vi "DCA Convert Limits Cluster.vi"(4 "Fields Names":string[](array[string]), 5 "Conversion":enum16{"Cluster - HTML", "HTML - Cluster"}(ring), 7 "Limits Key Array In":T6, 8 "Limits Cluster In":T1[](array[typedef])) -> (1 "Limits Cluster Out":T1[](array[typedef]), 2 "Limits HTML Out":string)   [LabVIEW 2011]
uses:
  ITK EXT/utils/keyedarr.llb/Keyed Array.ctl
  TypeDefs/DCA Limit.ctl
  TypeDefs/DCA Limit Quantity.ctl
  TypeDefs/DCA Limit Comparison.ctl
  TypeDefs/DCA Limit Operation.ctl
  Test Referential Limit.ctl
  ITK EXT/utils/strutil.llb/Case Matching.ctl
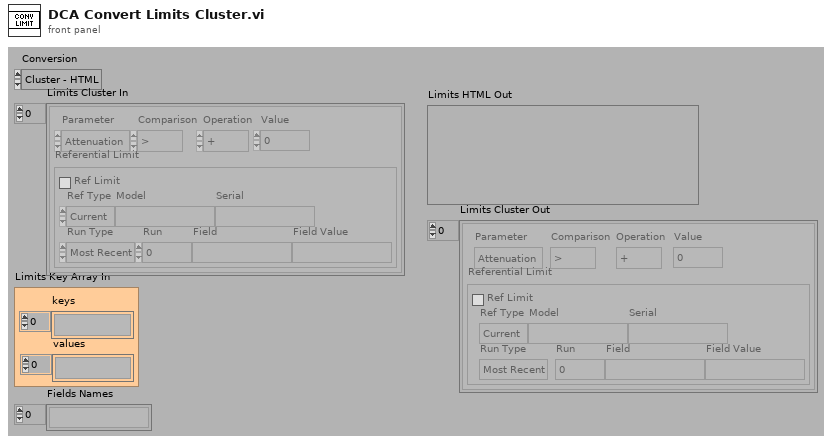
[diagram p1: front panel]
types:
  T1 = typedef "DCA Limit.ctl" = cluster{"Parameter":T2, "Comparison":T3, "Operation":T4, "Value":dbl, "Referential Limit":T5}
  T2 = typedef "DCA Limit Quantity.ctl" = enum16{"Attenuation", "Zin", "Zout", "R1", "R2", "R3", "Rab", "Rac", "Rbc"}
  T3 = typedef "DCA Limit Comparison.ctl" = enum16{">", ">=", "<", "<="}
  T4 = typedef "DCA Limit Operation.ctl" = enum16{"+", "-"}
  T5 = typedef "Test Referential Limit.ctl" = cluster{"Ref Limit":bool, "Ref Type":enum16{"Current", "Specify"}, "Model":string, "Serial":string, "Run Type":enum16{"Most Recent", "Run #", "Match Field"}, "Run":i32, "Field":string, "Field Value":string}
  T6 = typedef "Keyed Array.ctl" = cluster{"keys":string[], "values":string[]}
  T7 = typedef "Case Matching.ctl" = enum16{"a != A", "a == A", "system"}
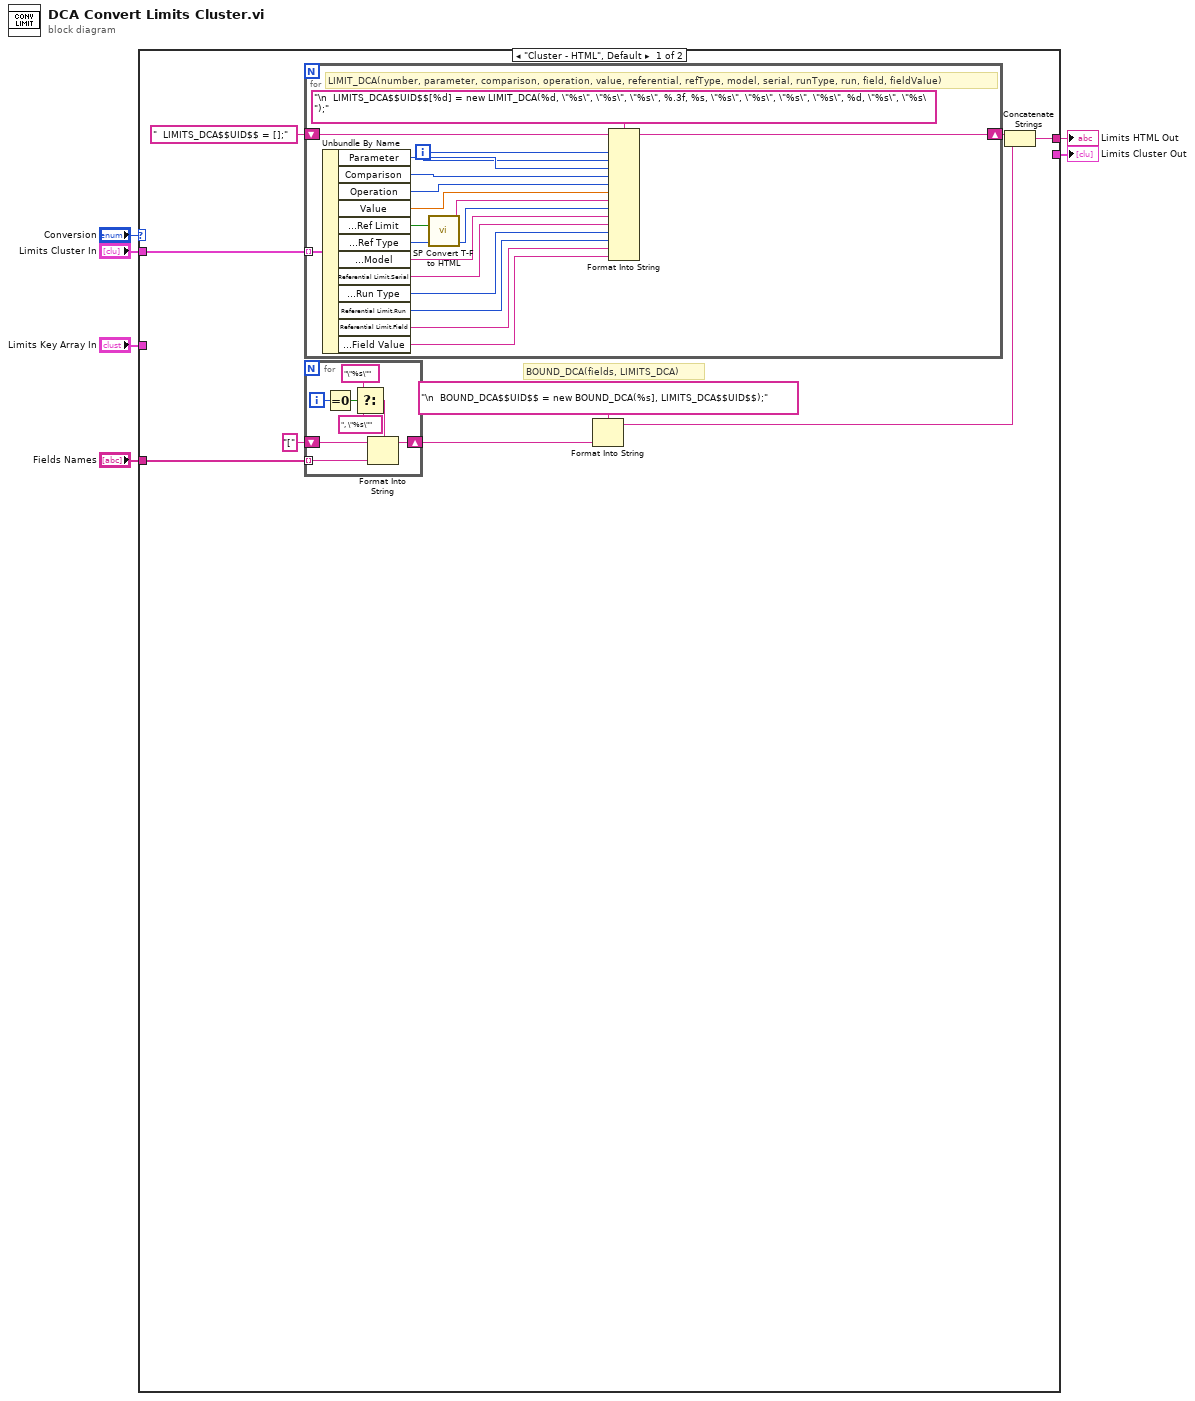
[diagram p0: block diagram]
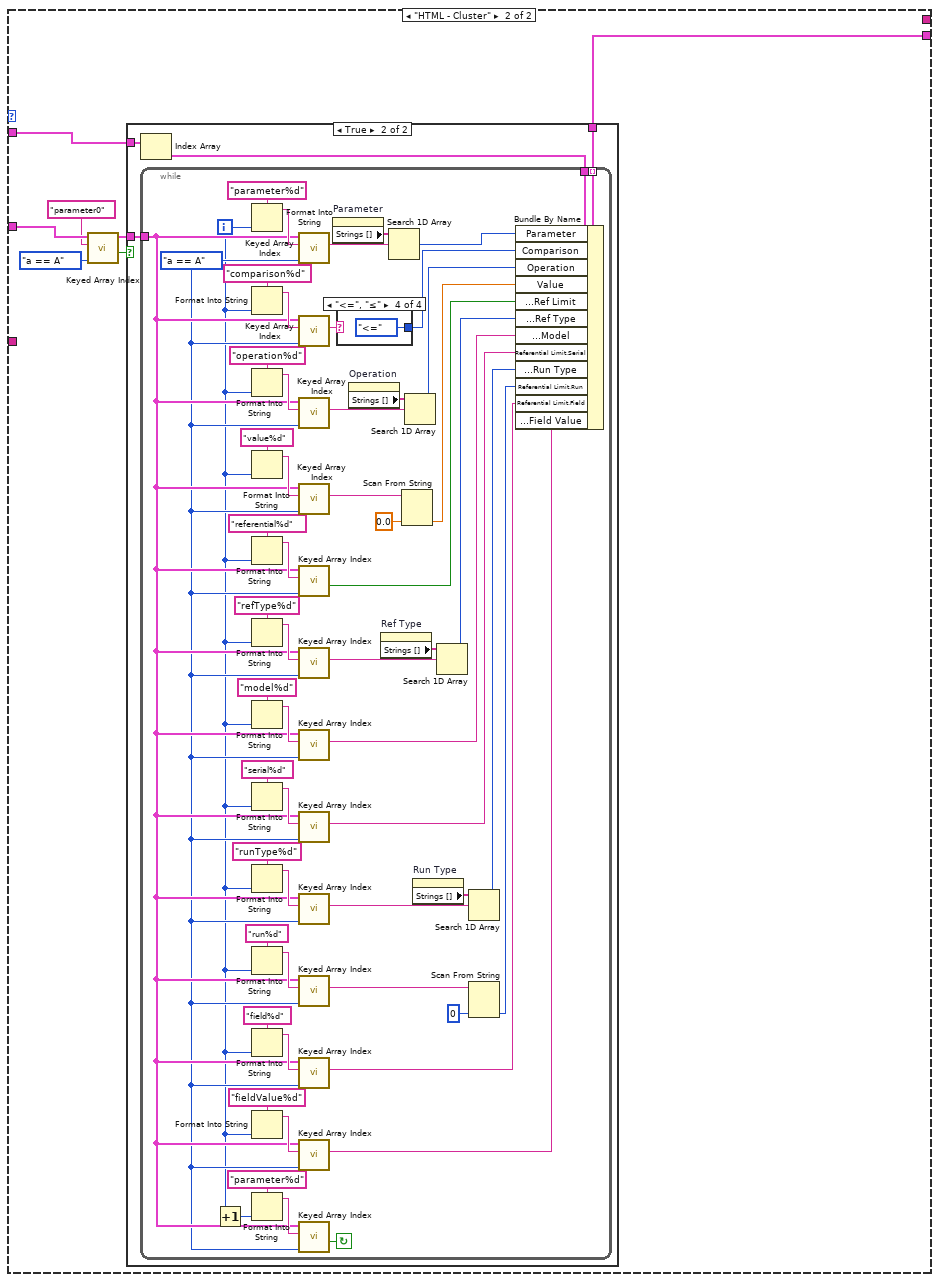
[diagram p2: hidden frame]
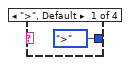
[diagram p4: hidden frame]
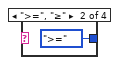
[diagram p5: hidden frame]
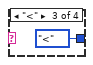
[diagram p6: hidden frame]
diagram:
  n1 = case shown="\"Cluster - HTML\", Default" "Conversion" {
    tunnel: "Limits Cluster In" -> [w15 w48]
    tunnel: "Limits Key Array In" -> [_ w46]
    tunnel: [w13 _] -> w3
    tunnel: [_ w47] -> w2
    tunnel: "Fields Names" -> [w10 _]
    frame "Cluster - HTML", Default {
      # "BOUND_DCA(fields, LIMITS_DCA)"
      n2 = for {
        tunnel: w15 -> [w41] mode=indexing
        shift-right: [w40] -> w12
        shift-left: "  LIMITS_DCA$$UID$$ = [];" ("format string") -> [w24]
        i -> [w25]
        # "LIMIT_DCA(number, parameter, comparison, operation, value, referential, refType, model, serial, runType, run, field, fieldValue)"
        n3 = Unbundle By Name(w41) -> ("Parameter"=w37:T2, "Comparison"=w36:T3, "Operation"=w35:T4, "Value"=w34:dbl, "Referential Limit.Ref Limit"=w38:bool, "Referential Limit.Ref Type"=w32:enum16{"Current", "Specify"}, "Referential Limit.Model"=w31:string, "Referential Limit.Serial"=w30:string, "Referential Limit.Run Type"=w29:enum16{"Most Recent", "Run #", "Match Field"}, "Referential Limit.Run"=w28:i32, "Referential Limit.Field"=w27:string, "Referential Limit.Field Value"=w26:string)
        n4 = call "SP Convert T-F to HTML.vi"("(T/F)"=w38) -> ("HTML (true/false)"=w33:string)  [unwired: 10 out]
        n5 = Format Into String(format string="\n  LIMITS_DCA$$UID$$[%d] = new LIMIT_DCA(%d, \"%s\", \"%s\", \"%s\", %.3f, %s, \"%s\", \"%s\", \"%s\", \"%s\", %d, \"%s\", \"%s\");", initial string=w24, w25, w25, w37, w36, w35, w34, w33, w32, w31, w30, w29, w28, w27, w26) -> (resulting string=w40:string)  [unwired: 1 in, 1 out]
      }
      n6 = for {
        shift-right: [w16] -> w8
        shift-left: "[" ("format string") -> [w23]
        tunnel: w10 -> [w17] mode=indexing
        i -> [w22]
        n7 = Equal To 0?(x=w22) -> (x = 0?=w21:bool)
        n8 = Select(t="\"%s\"" ("format string"), s=w21, f=", \"%s\"" ("format string")) -> (s? t:f=w18:string)
        n9 = Format Into String(format string=w18, initial string=w23, w17) -> (resulting string=w16:string)  [unwired: 1 in, 1 out]
      }
      n10 = Format Into String(format string="\n  BOUND_DCA$$UID$$ = new BOUND_DCA(%s], LIMITS_DCA$$UID$$);", w8) -> (resulting string=w7:string)  [unwired: 2 in, 1 out]
      n11 = Concatenate Strings(w12, w7) -> (w13:string)
    }
    frame "HTML - Cluster" {
      n12 = call "Keyed Array Index.vi"("case matching (sensitive)"=Case_Matching."a == A", "key"="parameter0", "array in"=w46) -> ("valid key"=w43:bool, "duplicate array"=w45:T6)  [unwired: 1 in, 2 out]
      n13 = case shown="True" w43 {
        tunnel: w48 -> [_ w52]
        tunnel: [_ w51] -> w47
        tunnel: w45 -> [_ w50]
        frame False {
        }
        frame True {
          n14 = Index Array(array=w52) -> (element=w49:T1)  [unwired: 1 in]
          n15 = while {
            tunnel: w49 -> [w110]
            tunnel: [w109] -> w51 mode=indexing
            tunnel: w50 -> [w59]
            i -> [w57]
            stop <- w67 continue-if-true
            w58 = Case_Matching."a == A" ("case matching (sensitive)")
            n16 = Increment(x=w57) -> (x+1=w68:i32)
            n17 = Format Into String(format string="parameter%d", w57) -> (resulting string=w107:string)  [unwired: 2 in, 1 out]
            n18 = Format Into String(format string="comparison%d", w57) -> (resulting string=w106:string)  [unwired: 2 in, 1 out]
            n19 = Format Into String(format string="operation%d", w57) -> (resulting string=w103:string)  [unwired: 2 in, 1 out]
            n20 = Format Into String(format string="value%d", w57) -> (resulting string=w60:string)  [unwired: 2 in, 1 out]
            n21 = Format Into String(format string="referential%d", w57) -> (resulting string=w102:string)  [unwired: 2 in, 1 out]
            n22 = Format Into String(format string="refType%d", w57) -> (resulting string=w99:string)  [unwired: 2 in, 1 out]
            n23 = Format Into String(format string="model%d", w57) -> (resulting string=w98:string)  [unwired: 2 in, 1 out]
            n24 = Format Into String(format string="serial%d", w57) -> (resulting string=w95:string)  [unwired: 2 in, 1 out]
            n25 = Format Into String(format string="runType%d", w57) -> (resulting string=w94:string)  [unwired: 2 in, 1 out]
            n26 = Format Into String(format string="run%d", w57) -> (resulting string=w91:string)  [unwired: 2 in, 1 out]
            n27 = Format Into String(format string="field%d", w57) -> (resulting string=w90:string)  [unwired: 2 in, 1 out]
            n28 = Format Into String(format string="fieldValue%d", w57) -> (resulting string=w87:string)  [unwired: 2 in, 1 out]
            n29 = Format Into String(format string="parameter%d", w68) -> (resulting string=w70:string)  [unwired: 2 in, 1 out]
            n30 = call "Keyed Array Index.vi"("case matching (sensitive)"=w58, "key"=w107, "array in"=w59) -> ("value"=w65:string)  [unwired: 1 in, 3 out]
            n31 = call "Keyed Array Index.vi"("case matching (sensitive)"=w58, "key"=w106, "array in"=w59) -> ("value"=w54:string)  [unwired: 1 in, 3 out]
            n32 = call "Keyed Array Index.vi"("case matching (sensitive)"=w58, "key"=w103, "array in"=w59) -> ("value"=w85:string)  [unwired: 1 in, 3 out]
            n33 = call "Keyed Array Index.vi"("case matching (sensitive)"=w58, "key"=w60, "array in"=w59) -> ("value"=w56:string)  [unwired: 1 in, 3 out]
            n34 = call "Keyed Array Index.vi"("case matching (sensitive)"=w58, "key"=w102, "array in"=w59) -> ("valid key"=w83:bool)  [unwired: 1 in, 3 out]
            n35 = call "Keyed Array Index.vi"("case matching (sensitive)"=w58, "key"=w99, "array in"=w59) -> ("value"=w81:string)  [unwired: 1 in, 3 out]
            n36 = call "Keyed Array Index.vi"("case matching (sensitive)"=w58, "key"=w98, "array in"=w59) -> ("value"=w79:string)  [unwired: 1 in, 3 out]
            n37 = call "Keyed Array Index.vi"("case matching (sensitive)"=w58, "key"=w95, "array in"=w59) -> ("value"=w78:string)  [unwired: 1 in, 3 out]
            n38 = call "Keyed Array Index.vi"("case matching (sensitive)"=w58, "key"=w94, "array in"=w59) -> ("value"=w76:string)  [unwired: 1 in, 3 out]
            n39 = call "Keyed Array Index.vi"("case matching (sensitive)"=w58, "key"=w91, "array in"=w59) -> ("value"=w74:string)  [unwired: 1 in, 3 out]
            n40 = call "Keyed Array Index.vi"("case matching (sensitive)"=w58, "key"=w90, "array in"=w59) -> ("value"=w71:string)  [unwired: 1 in, 3 out]
            n41 = call "Keyed Array Index.vi"("case matching (sensitive)"=w58, "key"=w87, "array in"=w59) -> ("value"=w55:string)  [unwired: 1 in, 3 out]
            n42 = call "Keyed Array Index.vi"("case matching (sensitive)"=w58, "key"=w70, "array in"=w59) -> ("valid key"=w67:bool)  [unwired: 1 in, 3 out]
            n43 = property on="Parameter" class="Enum (strict)"() -> ("Strings []"=w66:string[])  [unwired: 2 in, 2 out]
            n44 = case shown="\"<=\", \"≤\"" w54 {
              tunnel: [DCA_Limit_Comparison.">" ("Comparison") DCA_Limit_Comparison.">=" ("Comparison") DCA_Limit_Comparison."<" ("Comparison") DCA_Limit_Comparison."<=" ("Comparison")] -> w53
              frame ">", Default {
              }
              frame ">=", "≥" {
              }
              frame "<" {
              }
              frame "<=", "≤" {
              }
            }
            n45 = property on="Operation" class="Enum (strict)"() -> ("Strings []"=w86:string[])  [unwired: 2 in, 2 out]
            n46 = property on="Ref Type" class="Enum (strict)"() -> ("Strings []"=w82:string[])  [unwired: 2 in, 2 out]
            n47 = Search 1D Array(1D array=w66, element=w65) -> (index of element=w64:i32)  [unwired: 1 out]
            n48 = Scan From String(input string=w56, default 1=0.0 ("default value 1")) -> (output 1=w62:dbl)  [unwired: 3 in, 3 out]
            n49 = Search 1D Array(1D array=w86, element=w85) -> (index of element=w84:i32)  [unwired: 1 out]
            n50 = property on="Run Type" class="Enum (strict)"() -> ("Strings []"=w77:string[])  [unwired: 2 in, 2 out]
            n51 = Search 1D Array(1D array=w82, element=w81) -> (index of element=w80:i32)  [unwired: 1 out]
            n52 = Search 1D Array(1D array=w77, element=w76) -> (index of element=w75:i32)  [unwired: 1 out]
            n53 = Scan From String(input string=w74, default 1=0 ("default value 1")) -> (output 1=w73:i32)  [unwired: 3 in, 3 out]
            n54 = Bundle By Name(cluster=w110, "Parameter"=w64, "Comparison"=w53, "Operation"=w84, "Value"=w62, "Referential Limit.Ref Limit"=w83, "Referential Limit.Ref Type"=w80, "Referential Limit.Model"=w79, "Referential Limit.Serial"=w78, "Referential Limit.Run Type"=w75, "Referential Limit.Run"=w73, "Referential Limit.Field"=w71, "Referential Limit.Field Value"=w55) -> (w109:T1)
          }
        }
      }
    }
  }
  "Limits HTML Out" <- w3
  "Limits Cluster Out" <- w2
